vi "Apply Signal Names.vi"(8 "error in":errorcluster, 11 "2525 in":refnum<class "2525.lvclass">) -> (0 "error out":errorcluster, 3 "2525 out":refnum<class "2525.lvclass">)   [LabVIEW 2019, in "2525.lvlib" / "2525.lvclass"]
uses:
  Library/2525.lvclass
  C:/Users/Public/Documents/Development/builds/Instruments/SwitchMatrix.lvlibp/Library/SwitchMatrix.lvclass
  C:/Users/Public/Documents/Development/builds/Tools/Config.lvlibp/Config.lvclass
  builds/Instruments/SwitchMatrix.lvlibp/Accessors/Read Relay Name.vi
  builds/Tools/Config.lvlibp/Accessors/Read Device Signals.vi
  builds/Instruments/SwitchMatrix.lvlibp/Library/SwitchMatrix.lvclass
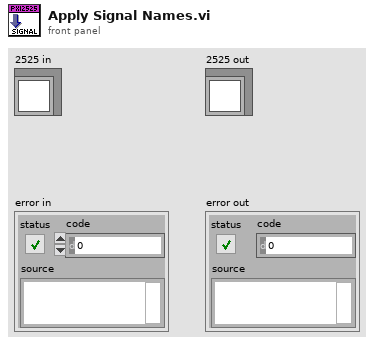
[diagram p1: front panel]
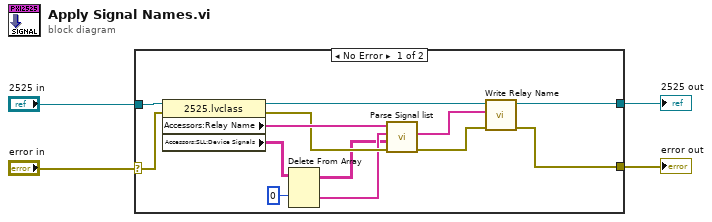
[diagram p0: block diagram]
diagram:
  n1 = case shown="No Error" "error in" {
    selector: "error in" -> [w16 w19]
    tunnel: [w13 w19] -> w3
    tunnel: [w14 w18] -> w1
    tunnel: "2525 in" -> [w17 w18]
    frame No Error {
      n2 = property class="2525.lvclass"(reference=w17, error in=w16) -> (reference out=w15:refnum<class "2525.lvclass">, error out=w9:errorcluster, "Accessors:Relay Name"=w10:string[], "Accessors:SLL:Device Signals"=w8:string[][])
      n3 = Delete From Array(array=w8, index (row)=0) -> (deleted portion=w6:string[], array with subset deleted=w5:string[][])  [unwired: 2 in]
      n4 = call "Parse Signal list.vi"("error in (no error)"=w9, "Signal List"=w5, "Headers"=w6, "Relay Names"=w10) -> ("error out"=w11:errorcluster, "Names"=w12:string[])  [unwired: 6 in]
      n5 = call "Write Relay Name.vi"("error in (no error)"=w11, "Relay Name"=w12, "SwitchMatrix in"=w15) -> ("error out"=w13:errorcluster, "SwitchMatrix out"=w14:refnum<class "2525.lvclass">)  [unwired: 7 in]
    }
    frame Error {
    }
  }
  "error out" <- w3
  "2525 out" <- w1
